vi "Compiled Code String.vi"(11 "ContainsCompiledCode":bool) -> (3 "Compiled Code String":string)   [LabVIEW 2023, in "VIDoc Printer.lvlib" / "VIDoc Printer.lvclass"]
doc: "Converts the Contains Compiled Code value into a printable String."
uses:
  VIDoc Printer.lvclass
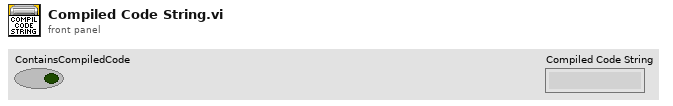
[diagram p1: front panel]
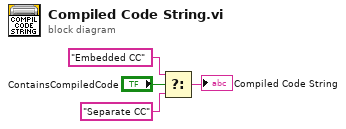
[diagram p0: block diagram]
diagram:
  n1 = Select(t="Embedded CC", s="ContainsCompiledCode", f="Separate CC") -> (s? t:f=→"Compiled Code String":string)
